vi "set_P_gas.vi"(0 "Run":bool, 1 "Gas In":bool, 2 "Active":bool, 3 "P_Gas Remote":bool=TRUE, 4 "H2 Flush":bool, 5 "P_Gas Flow":dbl) -> ()   [LabVIEW 2011]
uses:
  low_level_proc/globals.vi
  editor_lib/Flow_Globals.vi
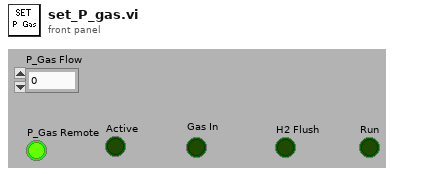
[diagram p1: front panel]
types:
  T1 = typedef "relaySpec.ctl" = cluster{"Card Index":u16, "Relay Index":u16}
  T2 = typedef "DA_Spec.ctl" = cluster{"Card Index":u16, "Channel Index":u16}
  T3 = typedef "AD_Spec.ctl" = u16
  T4 = cluster{"Relay Functions":cluster{"Remote":T1, "Active":T1, "Gas in":T1, "H2 flush":T1, "Run":T1}, "D/A Functions":cluster{"Flow":T2}, "Flow Range":cluster{"Flow (PGMFC1)":u16}, "A/D Functions":cluster{"Flow":T3}}
  T5 = cluster{"Remote":T1, "Active":T1, "Gas in":T1, "H2 flush":T1, "Run":T1}
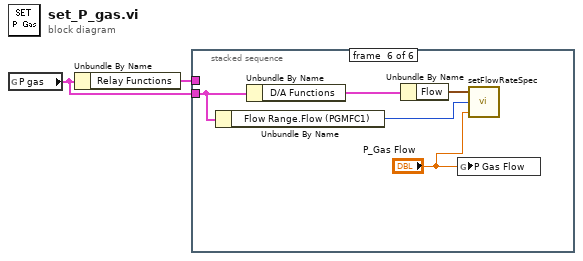
[diagram p0: block diagram]
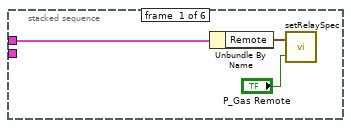
[diagram p2: hidden frame]
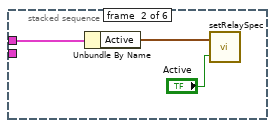
[diagram p3: hidden frame]
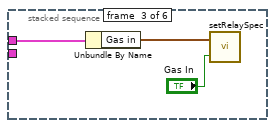
[diagram p4: hidden frame]
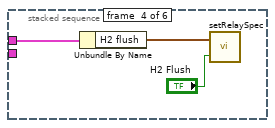
[diagram p5: hidden frame]
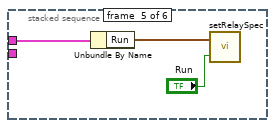
[diagram p6: hidden frame]
diagram:
  n1 = global read "globals.vi" "P gas"() -> (w1:T4)
  n2 = Unbundle By Name(w1) -> ("Relay Functions"=w2:T5)
  n3 = stacked-sequence {
    tunnel: w2 -> [w3 w6 w9 w12 w15 _]
    tunnel: w1 -> [_ _ _ _ _ w20]
    frame #0 {
      n4 = Unbundle By Name(w3) -> ("Remote"=w4:T1)
      n5 = call "setRelaySpec.vi"("Relay Status"="P_Gas Remote", "RelaySpec"=w4) -> ()  [unwired: 1 in]
    }
    frame #1 {
      n6 = Unbundle By Name(w6) -> ("Active"=w7:T1)
      n7 = call "setRelaySpec.vi"("Relay Status"="Active", "RelaySpec"=w7) -> ()  [unwired: 1 in]
    }
    frame #2 {
      n8 = Unbundle By Name(w9) -> ("Gas in"=w10:T1)
      n9 = call "setRelaySpec.vi"("Relay Status"="Gas In", "RelaySpec"=w10) -> ()  [unwired: 1 in]
    }
    frame #3 {
      n10 = Unbundle By Name(w12) -> ("H2 flush"=w13:T1)
      n11 = call "setRelaySpec.vi"("Relay Status"="H2 Flush", "RelaySpec"=w13) -> ()  [unwired: 1 in]
    }
    frame #4 {
      n12 = Unbundle By Name(w15) -> ("Run"=w16:T1)
      n13 = call "setRelaySpec.vi"("Relay Status"="Run", "RelaySpec"=w16) -> ()  [unwired: 1 in]
    }
    frame #5 {
      n14 = Unbundle By Name(w20) -> ("Flow Range.Flow (PGMFC1)"=w19:u16)
      n15 = Unbundle By Name(w20) -> ("D/A Functions"=w22:cluster{"Flow":T2})
      n16 = Unbundle By Name(w22) -> ("Flow"=w21:T2)
      n17 = global write "Flow_Globals.vi" "P Gas Flow"("P_Gas Flow") -> ()
      n18 = call "setFlowRateSpec.vi"("Flow Rate (sccm)"="P_Gas Flow", "Flow range Index"=w19, "D/A Card"=w21) -> ()  [unwired: 2 in]
    }
  }
